vi "Measurement-wise MN logic.vi"(11 "cluster":T2) -> (2 "Pause On Fail":bool, 3 "Measurement Details Array":T1(array[cluster]))   [LabVIEW 2019, in "Rack Controller.lvclass"]
uses:
  Rack Controller.lvclass
  Controls/Part Details_RC.ctl
  <vilib>/ActorFramework/Message Enqueuer/Message Enqueuer.lvclass
  Common/Controls/Camera Optics Diagnostics.ctl
  <vilib>/vision/Image Controls.llb/IMAQ Image.ctl
  Common/Controls/Camera Optics Diagnostics Result.ctl
  Inspection Statemachine/Controls/Result Cluster_SM.ctl
  Inspection Statemachine/Inspection Statemachine.lvclass
  Common/Controls/AllPartInfo.ctl
  Controls/Output Cluster_RC.ctl
  Controls/RC Local Data.ctl
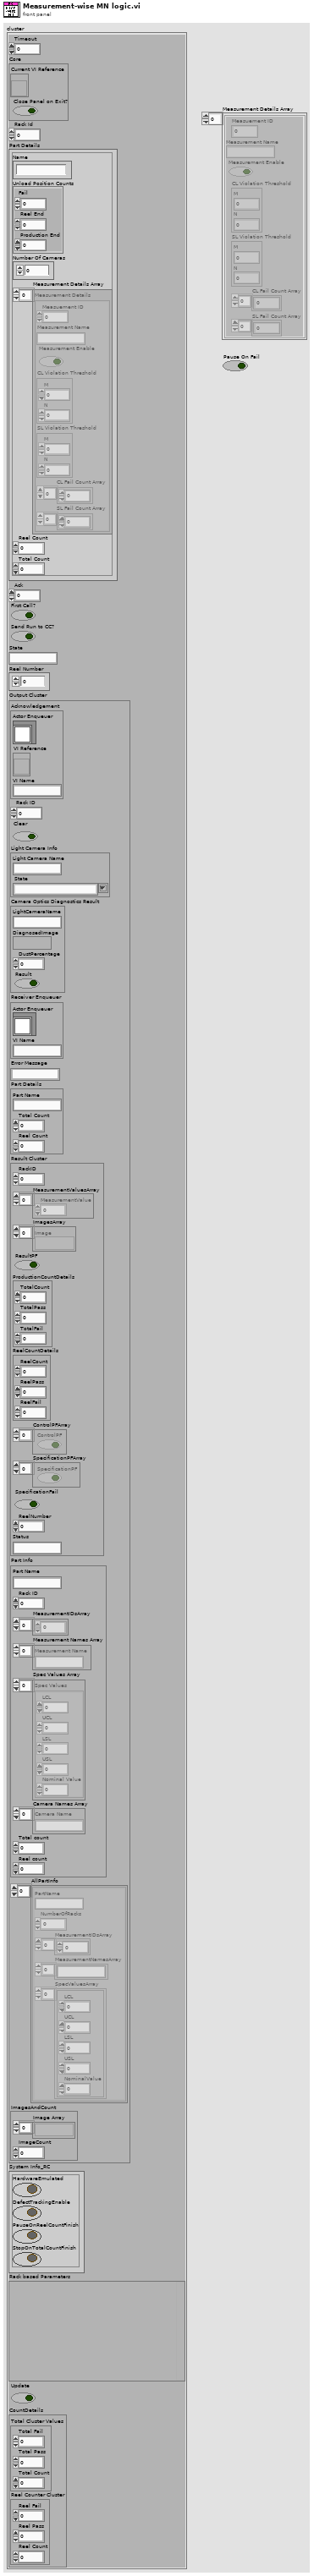
[diagram p1: front panel]
types:
  T1 = cluster{"Measuement ID":u16, "Measurement Name":string, "Measurement Enable":bool, "CL Violation Threshold":cluster{"M":u8, "N":u64}, "SL Violation Threshold":cluster{"M":u8, "N":u64}, "CL Fail Count Array":u64[], "SL Fail Count Array":u64[]}[]
  T2 = typedef "Rack Controller.lvclass/RC Local Data.ctl" = cluster{"Timeout":i32, "Core":cluster{"Current VI Reference":refnum<vi>, "Close Panel on Exit?":bool}, "Rack Id":u8, "Part Details":T3, "Ack":i32, "First Call?":bool, "Send Run to CC?":bool, "State":string, "Reel Number":u64, "Output Cluster":T4, "System Info_RC":cluster{"HardwareEmulated":bool, "DefectTrackingEnable":bool, "PauseOnReelCountFinish":bool, "StopOnTotalCountFinish":bool}, "Rack based Parameters":variant, "Update":bool, "CountDetails":cluster{"Total Cluster Values":cluster{"Total Fail":u64, "Total Pass":u64, "Total Count":u64}, "Reel Counter Cluster":cluster{"Reel Fail":u64, "Reel Pass":u64, "Reel Count":u64}}}
  T3 = typedef "Rack Controller.lvclass/Part Details_RC.ctl" = cluster{"Name":string, "Unload Position Counts":cluster{"Fail":u32, "Reel End":u32, "Production End":u32}, "Number Of Cameras":u8, "Measurement Details Array":cluster{"Measuement ID":u16, "Measurement Name":string, "Measurement Enable":bool, "CL Violation Threshold":cluster{"M":u8, "N":u64}, "SL Violation Threshold":cluster{"M":u8, "N":u64}, "CL Fail Count Array":u64[], "SL Fail Count Array":u64[]}[], "Reel Count":u64, "Total Count":u64}
  T4 = typedef "Rack Controller.lvclass/Output Cluster_RC.ctl" = cluster{"Acknowledgement":cluster{"Actor Enqueuer":refnum<class "Message Enqueuer.lvclass">, "VI Reference":refnum<vi>, "VI Name":string}, "Rack ID":u8, "Clear":bool, "Light Camera Info":T5, "Camera Optics Diagnostics Result":T6, "Receiver Enqueuer":cluster{"Actor Enqueuer":refnum<class "Message Enqueuer.lvclass">, "VI Name":string}, "Error Message":string, "Part Details":cluster{"Part Name":string, "Total Count":u64, "Reel Count":u64}, "Result Cluster":T8, "Part Info":cluster{"Part Name":string, "Rack ID":u8, "MeasurementIDsArray":u16[], "Measurement Names Array":string[], "Spec Values Array":cluster{"LCL":dbl, "UCL":dbl, "LSL":dbl, "USL":dbl, "Nominal Value":dbl}[], "Camera Names Array":string[], "Total count":u64, "Reel count":u64}, "AllPartInfo":T9, "ImagesAndCount":cluster{"Image Array":T7[], "ImageCount":u64}}
  T5 = typedef "Camera Optics Diagnostics.ctl" = cluster{"Light Camera Name":string, " State":string}
  T6 = typedef "Camera Optics Diagnostics Result.ctl" = cluster{"LightCameraName":string, "DiagnosedImage":T7, "DustPercentage":dbl, "Result":bool}
  T7 = typedef "IMAQ Image.ctl" = refnum<image>
  T8 = typedef "Inspection Statemachine.lvclass/Result Cluster_SM.ctl" = cluster{"RackID":u8, "MeasurementValuesArray ":dbl[], "ImagesArray":T7[], "ResultPF":bool, "ProductionCountDetails":cluster{"TotalFail":u64, "TotalPass":u64, "TotalCount":u64}, "ReelCountDetails":cluster{"ReelFail":u64, "ReelPass":u64, "ReelCount":u64}, "ControlPFArray":bool[], "SpecificationPFArray":bool[], "SpecificationFail":bool, "ReelNumber":u64, "Status":string}
  T9 = typedef "AllPartInfo.ctl" = cluster{"PartName":string, "NumberOfRacks":u8, "MeasurementIDsArray":u16[], "MeasurementNamesArray":string[], "SpecValuesArray":cluster{"LCL":dbl, "UCL":dbl, "LSL":dbl, "USL":dbl, "NominalValue":dbl}[]}[]
  T10 = cluster{"Measuement ID":u16, "Measurement Name":string, "Measurement Enable":bool, "CL Violation Threshold":cluster{"M":u8, "N":u64}, "SL Violation Threshold":cluster{"M":u8, "N":u64}, "CL Fail Count Array":u64[], "SL Fail Count Array":u64[]}
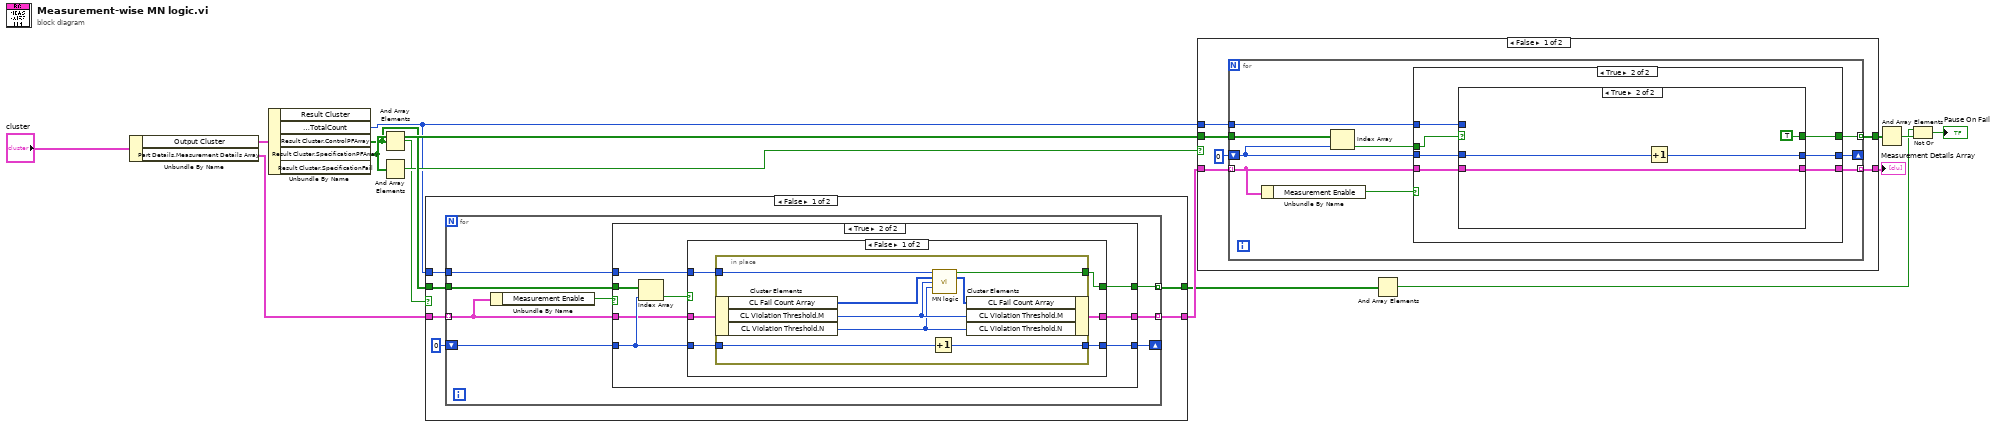
[diagram p0: block diagram]
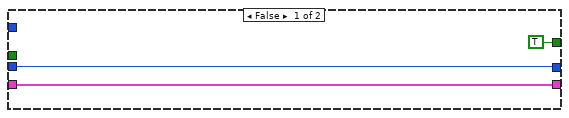
[diagram p2: hidden frame]
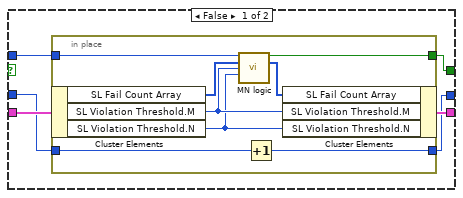
[diagram p3: hidden frame]
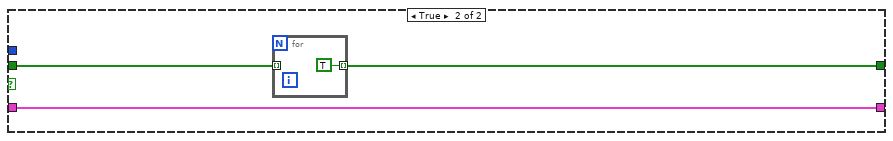
[diagram p4: hidden frame]
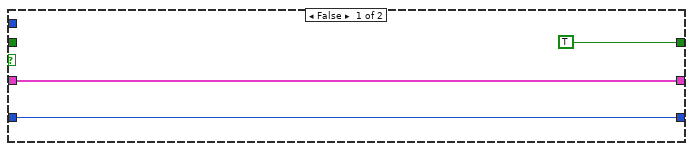
[diagram p5: hidden frame]
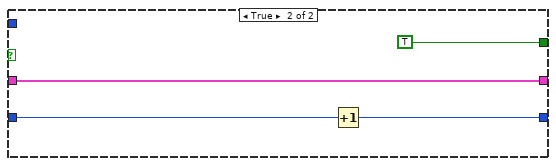
[diagram p6: hidden frame]
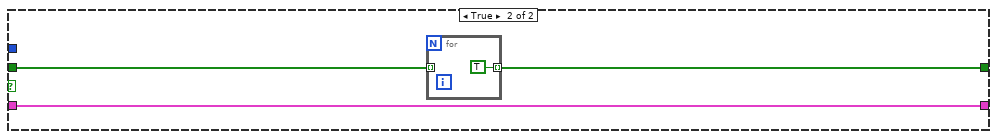
[diagram p7: hidden frame]
diagram:
  n1 = Unbundle By Name("cluster") -> ("Output Cluster"=w1:T4, "Part Details.Measurement Details Array"=w13:T1)
  n2 = Unbundle By Name(w1) -> ("Result Cluster.ProductionCountDetails.TotalCount"=w2:u64, "Result Cluster.ControlPFArray"=w10:bool[], "Result Cluster.SpecificationPFArray"=w11:bool[])  [unwired: 2 out]
  n3 = And Array Elements(Boolean array=w10) -> (logical AND=w3:bool)
  n4 = And Array Elements(Boolean array=w11) -> (logical AND=w4:bool)
  n5 = case shown="False" w3 {
    tunnel: w2 -> [w21 _]
    tunnel: w13 -> [w20 w61]
    tunnel: [w19 w59] -> w5
    tunnel: w10 -> [w17 w60]
    tunnel: [w18 w61] -> w14
    frame False {
      n6 = for {
        tunnel: w20 -> [w23] mode=indexing
        tunnel: w21 -> [w29]
        tunnel: [w28] -> w19 mode=indexing
        tunnel: [w27] -> w18 mode=indexing
        tunnel: w17 -> [w26]
        shift-right: [w25] -> _
        shift-left: 0 -> [w24]
        n7 = Unbundle By Name(w23) -> ("Measurement Enable"=w22:bool)
        n8 = case shown="True" w22 {
          tunnel: w29 -> [_ w40]
          tunnel: [TRUE ("Result Out") w39] -> w28
          tunnel: [w32 w38] -> w27
          tunnel: w26 -> [_ w37]
          tunnel: [w31 w35] -> w25
          tunnel: w24 -> [w31 w34]
          tunnel: w23 -> [w32 w33]
          frame False {
          }
          frame True {
            n9 = Index Array(array=w37, index=w34) -> (element=w36:bool)
            n10 = case shown="False" w36 {
              tunnel: w33 -> [w46 w58]
              tunnel: w40 -> [w45 _]
              tunnel: [w44 TRUE] -> w39
              tunnel: [w43 w58] -> w38
              tunnel: w34 -> [w42 w56]
              tunnel: [w41 w55] -> w35
              frame False {
                n11 = in-place {
                  in-place-border: w45 -> [w54]
                  in-place-border: [w49] -> w44
                  in-place-border: w42 -> [w48]
                  in-place-border: [w47] -> w41
                  n12 = in-place-cluster #1(w46) -> ("CL Fail Count Array"=w53:u64[], "CL Violation Threshold.M"=w51:u8, "CL Violation Threshold.N"=w50:u64)
                  n13 = Increment(x=w48) -> (x+1=w47:i32)
                  n14 = call "MN logic.vi"("Total Count"=w54, "Fail Count Array In"=w53, "M"=w51, "N"=w50) -> ("Result Out"=w49:bool, "Fail Count Array Out"=w52:u64[])  [unwired: 9 in, 1 out]
                  n15 = in-place-cluster #1("CL Fail Count Array"=w52, "CL Violation Threshold.M"=w51, "CL Violation Threshold.N"=w50) -> (w43:T10)
                }
              }
              frame True {
                n16 = Increment(x=w56) -> (x+1=w55:i32)
              }
            }
          }
        }
      }
    }
    frame True {
      n17 = for {
        tunnel: w60 -> [_] mode=indexing
        tunnel: [TRUE] -> w59 mode=indexing
      }
    }
  }
  n18 = case shown="False" w4 {
    tunnel: w2 -> [w68 _]
    tunnel: w14 -> [w67 w108]
    tunnel: [w66 w106] -> w6
    tunnel: w11 -> [w64 w107]
    tunnel: [w65 w108] -> w12
    frame False {
      n19 = for {
        tunnel: w67 -> [w73] mode=indexing
        tunnel: w68 -> [w77]
        tunnel: [w76] -> w66 mode=indexing
        tunnel: [w75] -> w65 mode=indexing
        tunnel: w64 -> [w74]
        shift-right: [w69] -> _
        shift-left: 0 -> [w70]
        n20 = Unbundle By Name(w73) -> ("Measurement Enable"=w72:bool)
        n21 = Index Array(array=w74, index=w70) -> (element=w71:bool)
        n22 = case shown="True" w72 {
          tunnel: w77 -> [_ w87]
          tunnel: [TRUE ("Result Out") w86] -> w76
          tunnel: [w80 w85] -> w75
          tunnel: w73 -> [w80 w84]
          tunnel: w71 -> [_ w83]
          tunnel: w70 -> [w78 w82]
          tunnel: [w78 w81] -> w69
          frame False {
          }
          frame True {
            n23 = case shown="True" w83 {
              tunnel: w84 -> [w93 w104]
              tunnel: w87 -> [w92 _]
              tunnel: [w91 TRUE ("Result Out")] -> w86
              tunnel: [w90 w104] -> w85
              tunnel: w82 -> [w89 w103]
              tunnel: [w88 w102] -> w81
              frame False {
                n24 = in-place {
                  in-place-border: w92 -> [w101]
                  in-place-border: [w96] -> w91
                  in-place-border: w89 -> [w95]
                  in-place-border: [w94] -> w88
                  n25 = in-place-cluster #2(w93) -> ("SL Fail Count Array"=w100:u64[], "SL Violation Threshold.M"=w98:u8, "SL Violation Threshold.N"=w97:u64)
                  n26 = call "MN logic.vi"("Total Count"=w101, "Fail Count Array In"=w100, "M"=w98, "N"=w97) -> ("Result Out"=w96:bool, "Fail Count Array Out"=w99:u64[])  [unwired: 9 in, 1 out]
                  n27 = Increment(x=w95) -> (x+1=w94:i32)
                  n28 = in-place-cluster #2("SL Fail Count Array"=w99, "SL Violation Threshold.M"=w98, "SL Violation Threshold.N"=w97) -> (w90:T10)
                }
              }
              frame True {
                n29 = Increment(x=w103) -> (x+1=w102:i32)
              }
            }
          }
        }
      }
    }
    frame True {
      n30 = for {
        tunnel: [TRUE] -> w106 mode=indexing
        tunnel: w107 -> [_] mode=indexing
      }
    }
  }
  "Measurement Details Array" <- w12
  n31 = And Array Elements(Boolean array=w5) -> (logical AND=w7:bool)
  n32 = And Array Elements(Boolean array=w6) -> (logical AND=w8:bool)
  n33 = Not Or(1:w8, 2:w7) -> (0:→"Pause On Fail":bool)
